vi "Octal to Hexa Decimal.vi"(11 "Octal Number":i64 format="%o") -> (3 "Hexa Decimal Number":i64 format="%x")   [LabVIEW 2020]
doc: "This VI will convert Octal Values to Hexa Decimal Values."
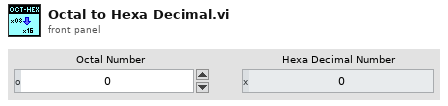
[diagram p1: front panel]
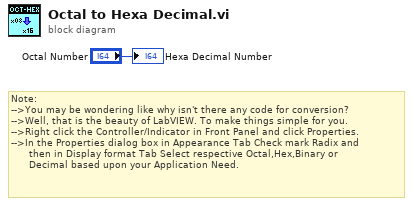
[diagram p0: block diagram]
diagram:
  # "Note: \n-->You may be wondering like why isn't there any code for conversion?\n-->Well, that is the beauty of LabVIEW. To make things simple for you.\n-->Right click the Controller/Indicator in Front Panel and click Properties.\n-->In the Properties dialog box in Appearance Tab Check mark Radix and \n      then in Display format Tab Select respective Octal,Hex,Binary or\n      Decimal based upon your Application Need."
  "Hexa Decimal Number" <- "Octal Number"
